vi "Read (Multiple Points).vi"(0 "VISA resource name":refnum<visa-resource-name>, 1 "Buffer Elements":string="READ", 5 "Timeout (10000 ms)":i32=10000 format="%#.6g", 7 "Start Index (1)":u32=1, 9 "End Index (1)":u32=1, 11 "error in (no error)":errorcluster, 12 "Buffer Name (defbuffer1)":string="defbuffer1") -> (4 "VISA resource name out":refnum<visa-resource-name>, 6 "Data out":string, 15 "error out":errorcluster)   [LabVIEW 2022 SP3, in "Keithley 2450.lvlib"]
doc: "Initiates an acquisition and returns the raw data gathered from the instrument.\n\nBuffer Element can be a single parameter or multiple parameters.Parameters have to be separated by comma followed by space.(eg - READ, SEC, DATE)"
uses:
  C:/Users/Public/OneDrive/Desktop/test_save_lv22/Close.vi/Close Folder/Users/Public/OneDrive/Desktop/Keithley_2450_2470_1_4_0_LV2015_NewReadme2_2450-LV2015-1.4.0/Keithley 2450/Keithley 2450.lvlib
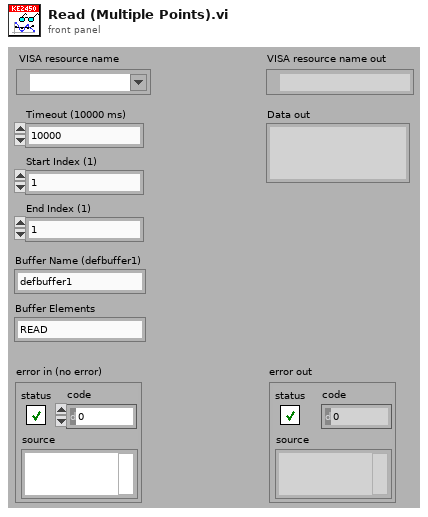
[diagram p1: front panel]
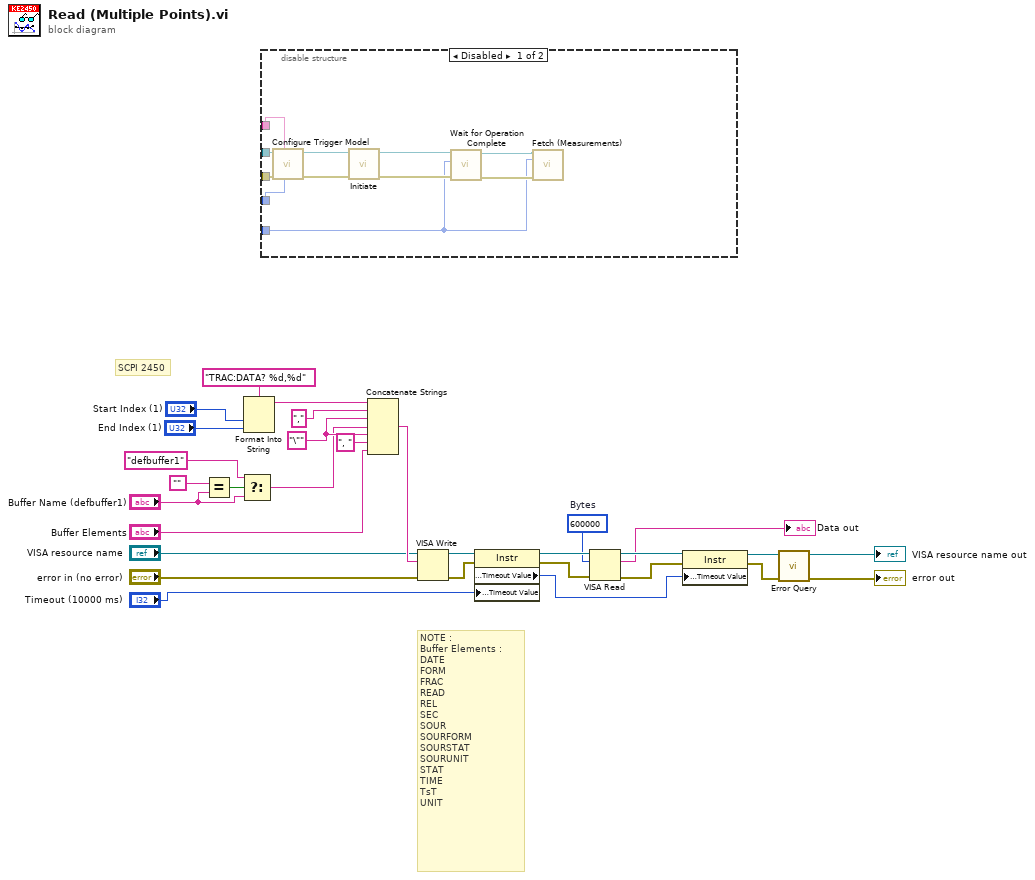
[diagram p0: block diagram]
diagram:
  w15 = "\""
  w21 = u32 600000  # Bytes
  # "NOTE :\nBuffer Elements :\nDATE\nFORM\nFRAC\nREAD\nREL\nSEC\nSOUR\nSOURFORM\nSOURSTAT\nSOURUNIT\nSTAT\nTIME\nTsT\nUNIT"
  # "SCPI 2450"
  n1 = Equal?(x="", y="Buffer Name (defbuffer1)") -> (x = y?=w17:bool)
  n2 = Select(t="defbuffer1", s=w17, f="Buffer Name (defbuffer1)") -> (s? t:f=w14:string)
  n3 = Format Into String(format string="TRAC:DATA? %d,%d" ("Fetch Measurement"), "Start Index (1)", "End Index (1)") -> (resulting string=w4:string)  [unwired: 2 in, 1 out]
  n4 = disable-structure shown="Disabled" {
    disable-tunnel: _ -> [w37 _]
    disable-tunnel: _ -> [w36 _]
    disable-tunnel: _ -> [w35 _]
    disable-tunnel: _ -> [w34 _]
    disable-tunnel: _ -> [w31 _]
    frame Disabled {
      n5 = call <instrlib>:"Configure Trigger Model.vi"("Trigger Count (1)"=w36, "Buffer Name (defbuffer1)"=w31, "error in (no error)"=w34, "VISA resource name"=w35) -> ("error out"=w32:errorcluster, "VISA resource name out"=w33:refnum<visa-resource-name>)  [unwired: 6 in]
      n6 = call <instrlib>:"Initiate.vi"("error in (no error)"=w32, "VISA resource name"=w33) -> ("error out"=w40:errorcluster, "VISA resource name out"=w41:refnum<visa-resource-name>)  [unwired: 8 out]
      n7 = call <instrlib>:"Wait for Operation Complete.vi"("error in (no error)"=w40, "Timeout (10000 ms)"=w37, "VISA resource name"=w41) -> ("error out"=w39:errorcluster, "VISA resource name out"=w38:refnum<visa-resource-name>)  [unwired: 7 out]
      n8 = call <instrlib>:"Fetch (Measurements).vi"("VISA resource name"=w38, "Timeout (10000 ms)"=w37, "error in (no error)"=w39) -> ()  [unwired: 2 in, 11 out]
    }
    frame Enabled {
    }
  }
  n9 = Concatenate Strings(w4, "," ("string"), w15, w14, w15, ", " ("string"), "Buffer Elements") -> (w28:string)
  n10 = VISA Write(VISA resource name="VISA resource name", write buffer=w28, error in (no error)="error in (no error)") -> (VISA resource name out=w19:refnum<visa-resource-name>, error out=w27:errorcluster)  [unwired: 1 out]
  n11 = property class="Instr"(reference=w19, error in=w27, "General Settings:Timeout Value"="Timeout (10000 ms)") -> (reference out=w26:refnum<visa-resource-name>, error out=w25:errorcluster, "General Settings:Timeout Value"=w22:u32)
  n12 = VISA Read(VISA resource name=w26, byte count=w21, error in (no error)=w25) -> (VISA resource name out=w24:refnum<visa-resource-name>, read buffer=→"Data out":string, error out=w23:errorcluster)  [unwired: 1 out]
  n13 = property class="Instr"(reference=w24, error in=w23, "General Settings:Timeout Value"=w22) -> (reference out=w13:refnum<visa-resource-name>, error out=w12:errorcluster)
  n14 = call "Error Query.vi"("error in (no error)"=w12, "VISA resource name"=w13) -> ("error out"=→"error out":errorcluster, "VISA resource name out"=→"VISA resource name out":refnum<visa-resource-name>)  [unwired: 8 out]
